vi "Brewster Angle Analysis.vi"(0 "Open File":path, 5 "q Starting   2":dbl, 9 "q Final":dbl, 11 "Do BA Analysis":bool) -> (3 "No. de datos":i32, 4 "qR":dbl, 6 "Curve width":dbl format="%#.3g", 8 "q  Middle":dbl, 10 "Minimun Intensity":dbl, 13 "Reflective Index":dbl, 14 "Curve":cluster{"EJE X":dbl[], dbl[]}(graph), 15 "Maximum Intensity":dbl)   [LabVIEW 2025, in "Control de MaP.lvlib"]
uses:
  Control de MaP.lvlib
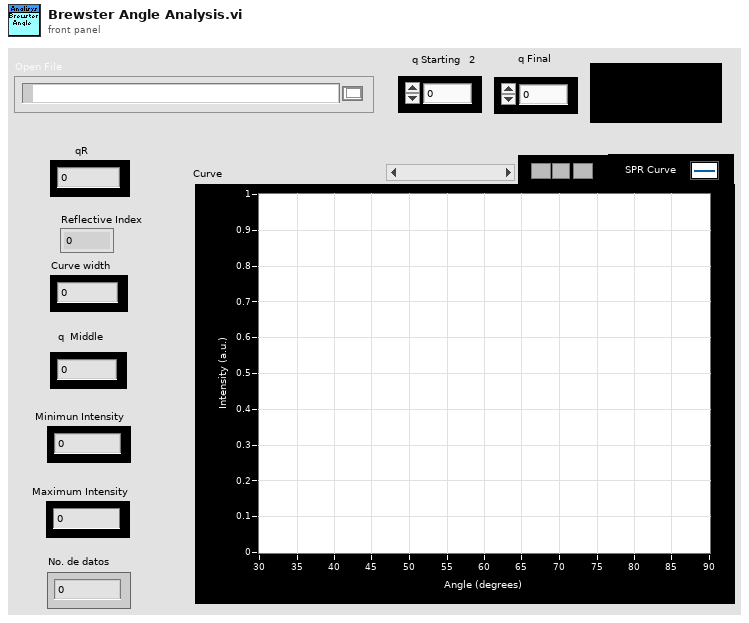
[diagram p1: front panel]
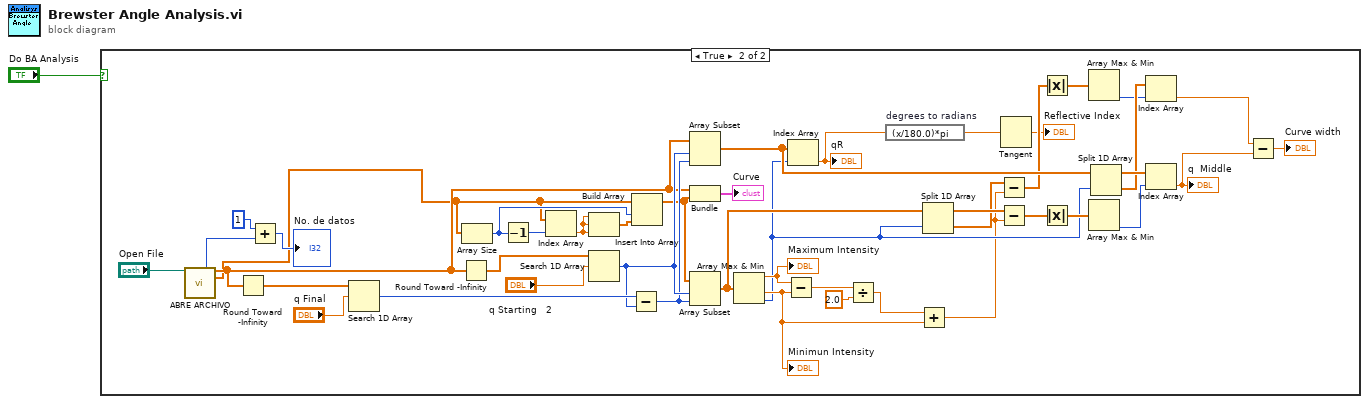
[diagram p0: block diagram]
diagram:
  n1 = case shown="True" "Do BA Analysis" {
    frame False {
    }
    frame True {
      n2 = call "ABRE ARCHIVO.vi"("File Path Control"="Open File") -> ("Número de datos"=w8:i32, "EJE X"=w10:dbl[], "EJE Y"=w2:dbl[])  [unwired: 9 in, 3 out]
      n3 = Round Toward -Infinity(1:w10) -> (0:w11:dbl[])
      n4 = Add(x=1, y=w8) -> (x+y=→"No. de datos":i32)
      n5 = Search 1D Array(1D array=w11, element="q Final") -> (index of element=w44:i32)  [unwired: 1 in]
      n6 = Round Toward -Infinity(1:w10) -> (0:w9:dbl[])
      n7 = Array Size(array=w2) -> (size(s)=w41:i32)
      n8 = Decrement(x=w41) -> (x-1=w43:i32)
      n9 = Index Array(array=w2, index=w43) -> (element=w42:dbl)
      n10 = Build Array(w42, w42, w42) -> (w40:dbl[])
      n11 = Search 1D Array(1D array=w9, element="q Starting   2") -> (index of element=w39:i32)  [unwired: 1 in]
      n12 = Subtract(x=w44, y=w39) -> (x-y=w38:i32)
      n13 = Insert Into Array(array=w2, index=w41, new element=w40) -> (w37:dbl[])
      n14 = Array Subset(array=w10, index=w39, length=w38) -> (w26:dbl[])
      n15 = Bundle("EJE X"=w10, "EJE Y"=w37) -> (→"Curve":cluster{"EJE X":dbl[], "EJE Y":dbl[]})  [unwired: 1 in]
      n16 = Array Subset(array=w37, index=w39, length=w38) -> (w30:dbl[])
      n17 = Array Max & Min(array=w30) -> (max value=w35:dbl, min value=w31:dbl, min index (indices)=w22:i32)  [unwired: 1 out]
      "Minimun Intensity" <- w31
      "Maximum Intensity" <- w35
      n18 = Subtract(x=w35, y=w31) -> (x-y=w34:dbl)
      n19 = Index Array(array=w26, index=w22) -> (element=w4:dbl)
      "qR" <- w4
      n20 = Divide(x=w34, y=2.0) -> (x/y=w32:dbl)
      n21 = expression code="(x/180.0)*pi" "degrees to radians"(w4) -> (w3:dbl)
      n22 = Add(x=w32, y=w31) -> (x+y=w18:dbl)
      n23 = Split 1D Array(array=w30, index=w22) -> (first subarray=w29:dbl[], second subarray=w19:dbl[])
      n24 = Subtract(x=w19, y=w18) -> (x-y=w20:dbl[])
      n25 = Subtract(x=w29, y=w18) -> (x-y=w28:dbl[])
      n26 = Tangent(1:w3) -> (0:→"Reflective Index":dbl)
      n27 = Absolute Value(x=w20) -> (abs(x)=w21:dbl[])
      n28 = Absolute Value(x=w28) -> (abs(x)=w27:dbl[])
      n29 = Array Max & Min(array=w21) -> (min index (indices)=w17:i32)  [unwired: 3 out]
      n30 = Array Max & Min(array=w27) -> (min index (indices)=w24:i32)  [unwired: 3 out]
      n31 = Split 1D Array(array=w26, index=w22) -> (first subarray=w25:dbl[], second subarray=w23:dbl[])
      n32 = Index Array(array=w23, index=w17) -> (element=w16:dbl)
      n33 = Index Array(array=w25, index=w24) -> (element=w15:dbl)
      "q  Middle" <- w15
      n34 = Subtract(x=w16, y=w15) -> (x-y=→"Curve width":dbl)
    }
  }
